vi "FormulaCleanup.vi"(0 "__args":T2) -> (1 "__return":cluster{"destinations":u32[][]}, 2 "__errStatus":bool, 3 "__errCode":i32, 4 "__errSource":string)   [LabVIEW 2013]
uses:
  <vilib>/Utility/miscctls.llb/LVRectTypeDef.ctl
panel:
  out "destinations":u32[][](array[numeric])
  out "st":i32[](array[numeric])
  out "Ntot":i32
  out "input_flag":i16[](array[numeric])
  out "N_in_out":i32[](array[numeric])
  out "s":i32[](array[numeric])
  in  "edge":i32 caption="0:L/R, 1:T/B"
  out "terminal_names":string[](array[string])
  out "terminal_rects":u32[][](array[numeric])
  out "formula_rect":T1
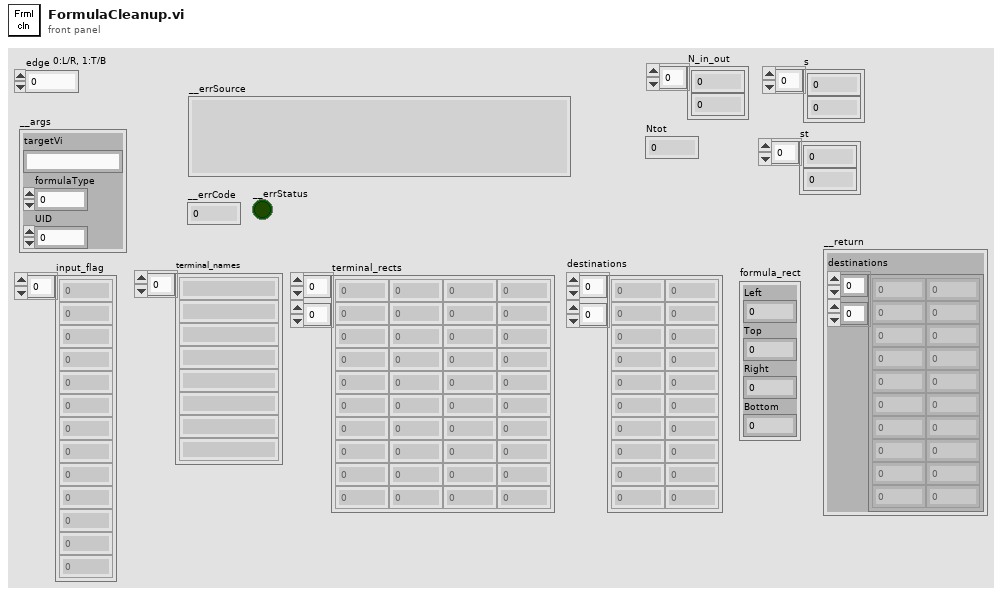
[diagram p1: front panel]
types:
  T1 = typedef "LVRectTypeDef.ctl" = cluster{"Left":i16, "Top":i16, "Right":i16, "Bottom":i16}
  T2 = cluster{"targetVi":string, "formulaType":i32, "UID":i32}
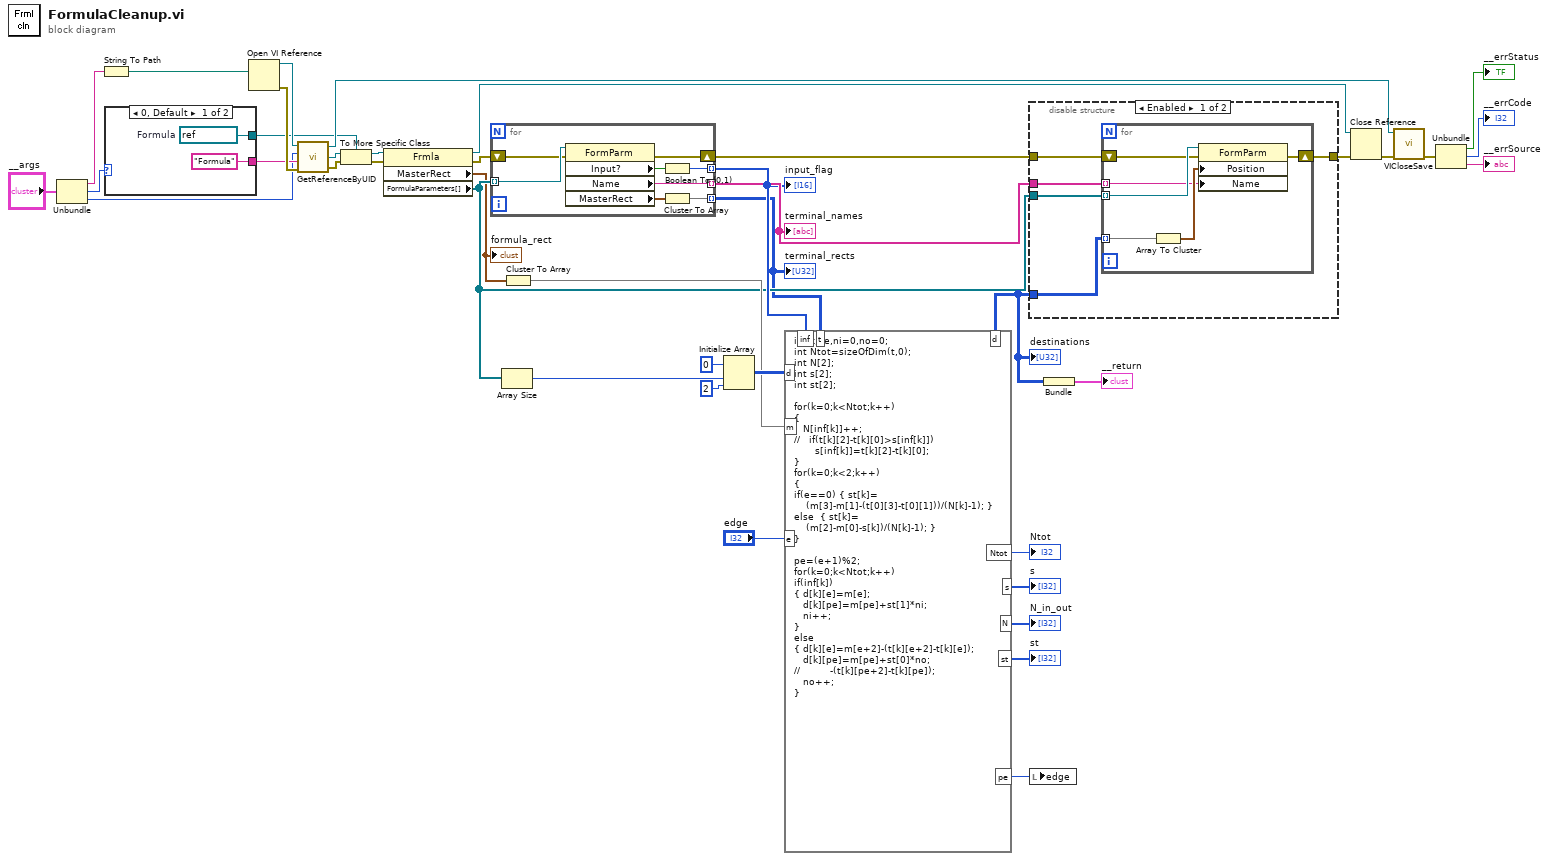
[diagram p0: block diagram]
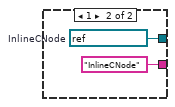
[diagram p3: hidden frame]
diagram:
  n1 = Unbundle("__args") -> ("targetVi"=w35:string, "formulaType"=w25:i32, "UID"=w26:i32)
  n2 = String To Path(string=w35) -> (path=w37:path)
  n3 = case shown="0, Default" w25 {
    tunnel: [w43 w45] -> w28
    tunnel: ["Formula" ("objectClass") "InlineCNode" ("objectClass")] -> w27
    frame 0, Default {
      w43 = refnum<vi> refnum  # Formula
    }
    frame 1 {
      w45 = refnum<vi> refnum  # InlineCNode
    }
  }
  n4 = Open VI Reference(vi path=w37) -> (vi reference=w34:refnum<vi>, error out=w36:errorcluster)  [unwired: 5 in]
  n5 = call "GetReferenceByUID.vi"("error in (no error)"=w36, "objectClass"=w27, "UID"=w26, "targetVI"=w34) -> ("error out"=w33:errorcluster, "refNum"=w32:refnum<vi>, "dup targetVI"=w30:refnum<vi>)
  n6 = To More Specific Class(target class=w28, reference=w32, error in=w33) -> (specific class reference=w9:refnum<vi>, error out=w8:errorcluster)
  n7 = property class="Frmla"(reference=w9, error in=w8) -> (reference out=w4:refnum<vi>, error out=w11:errorcluster, "MasterRect"=w2:T1, "FormulaParameters[]"=w3:refnum<vi>[])
  "formula_rect" <- w2
  n8 = for {
    tunnel: w3 -> [w53] mode=indexing
    tunnel: [w51] -> w1 mode=indexing
    tunnel: [w50] -> w10 mode=indexing
    tunnel: [w48] -> w5 mode=indexing
    shift-right: [w46] -> w7
    shift-left: w11 -> [w47]
    n9 = property class="FormParm"(reference=w53, error in=w47) -> (error out=w46:errorcluster, "Input?"=w49:bool, "Name"=w50:string, "MasterRect"=w52:T1)  [unwired: 1 out]
    n10 = Boolean To (0,1)(Boolean=w49) -> (0, 1=w48:i16)
    n11 = Cluster To Array(cluster=w52) -> (array=w51:i16[])
  }
  "terminal_rects" <- w1
  "terminal_names" <- w10
  "input_flag" <- w5
  n12 = Array Size(array=w3) -> (size(s)=w22:i32)
  n13 = Cluster To Array(cluster=w2) -> (array=w6:i16[])
  n14 = Initialize Array(u32 0 ("Width"), w22, 2 ("dimension size")) -> (w20:u32[][])
  n15 = formula code="int k,pe,ni=0,no=0;\nint Ntot=sizeOfDim(t,0);\nint N[2];\nint s[2];\nint st[2];\n\nfor(k=0;k<Ntot;k++)\n{\n   N[inf[k]]++;\n//   if(t[k][2]-t[k][0]>s[inf[k]])\n       s[inf[k]]=t[k][2]-t[k][0];\n}\nfor(k=0;k<2;k++)\n{\nif(e==0) { st[k]=\n    (m[3]-m[1]-(t[0][3]-t[0][1]))/(N[k]-1); }\nelse  { st[k]=\n    (m[2]-m[0]-s[k])/(N[k]-1); }\n}\n\npe=(e+1)%2;\nfor(k=0;k<Ntot;k++)\nif(inf[k])\n{ d[k][e]=m[e];\n   d[k][pe]=m[pe]+st[1]*ni;\n   ni++;\n}\nelse\n{ d[k][e]=m[e+2]-(t[k][e+2]-t[k][e]);\n   d[k][pe]=m[pe]+st[0]*no; \n//          -(t[k][pe+2]-t[k][pe]);\n   no++;\n}"("m"=w6, "t"=w1, "d"=w20, "e"="edge", "inf"=w5) -> ("d"=w14:u32[][], "s"=→"s":i32[], "N"=→"N_in_out":i32[], "Ntot"=→"Ntot":i32, "st"=→"st":i32[], "pe"=w12:i32)
  "destinations" <- w14
  n16 = disable-structure shown="Enabled" {
    disable-tunnel: w14 -> [w58 _]
    disable-tunnel: w3 -> [w57 _]
    disable-tunnel: w7 -> [w56 w65]
    disable-tunnel: [w55 w65] -> w17
    disable-tunnel: w10 -> [w54 _]
    frame Enabled {
      n17 = for {
        tunnel: w58 -> [w63] mode=indexing
        tunnel: w57 -> [w62] mode=indexing
        shift-right: [w60] -> w55
        shift-left: w56 -> [w61]
        tunnel: w54 -> [w59] mode=indexing
        n18 = Array To Cluster(array=w63) -> (cluster=w64:cluster{"d[0]":u32, "d[1]":u32})
        n19 = property class="FormParm"(reference=w62, error in=w61, "Position"=w64, "Name"=w59) -> (error out=w60:errorcluster)  [unwired: 1 out]
      }
    }
    frame Disabled {
    }
  }
  n20 = local write "edge"(w12) -> ()
  n21 = Bundle("d"=w14) -> (→"__return":cluster{"d":u32[][]})  [unwired: 1 in]
  n22 = Close Reference(reference=w4, error in (no error)=w17) -> (error out=w29:errorcluster)
  n23 = call "VICloseSave.vi"("error in (no error)"=w29, "VI in"=w30) -> ("error out"=w31:errorcluster)  [unwired: 9 in]
  n24 = Unbundle(w31) -> ("status"=→"__errStatus":bool, "code"=→"__errCode":i32, "source"=→"__errSource":string)
